vi "Online_Target_2.vi"   [LabVIEW 2021]
uses:
  Model_Updating_Classes/DROPBEAR_Model_Updating/DROPBEAR_Model_Updating.lvclass
types:
  T1 = cluster{"beam_length":dbl, "youngs_modulus":dbl, "torsion_spring":dbl, "beam_height":dbl, "beam_width":dbl, "beam_density":dbl, "number_of_FEA_nodes":i32, "accelerometer_mass":dbl}
  T2 = cluster{"Frequency KF":bool, "Pinned State KF":bool, "FFT Bounding":bool, "Filter Constants Frequency":cluster{"Measurement Variance":dbl, "State Variance":dbl, "Threshold":dbl}, "Filter Constants Position":cluster{"Measurement Variance":dbl, "State Variance":dbl, "Threshold":dbl}, "Moving Window Size":i32, "Time Series buffer":dbl, "Record Time Series Data":bool, "Record Moving Window Data":bool, "Record Online Error Metrics ":bool, "Record Statistics":bool}
  T3 = cluster{"Eigensolver ":enum16{"LabVIEW Cholesky", "LabVIEW General", "LabVIEW Inverse", "LEMP"}, "Models Forcasted":i32, "Max Roller Velocity":dbl, "Max Roller Position Percent":dbl, "Min Roller Position Percent":dbl}
  T4 = cluster{"Dataset":string, "Resample Method":enum16{"Recorded", "Auto Resample", "Custom Resample"}}
  T5 = cluster{"Modeling Parameters input controls":cluster{"beam_length":dbl, "youngs_modulus":dbl, "torsion_spring":dbl, "beam_height":dbl, "beam_width":dbl, "beam_density":dbl, "number_of_FEA_nodes":i32, "accelerometer_mass":dbl}, "Mockbear input controls":cluster{"Dataset":string, "Resample Method":enum16{"Recorded", "Auto Resample", "Custom Resample"}}, "Simulation Parameters input controls":cluster{"Eigensolver ":enum16{"LabVIEW Cholesky", "LabVIEW General", "LabVIEW Inverse", "LEMP"}, "Models Forcasted":i32, "Max Roller Velocity":dbl, "Max Roller Position Percent":dbl, "Min Roller Position Percent":dbl}, "Program Controls":cluster{"Frequency KF":bool, "Pinned State KF":bool, "FFT Bounding":bool, "Filter Constants Frequency":cluster{"Measurement Variance":dbl, "State Variance":dbl, "Threshold":dbl}, "Filter Constants Position":cluster{"Measurement Variance":dbl, "State Variance":dbl, "Threshold":dbl}, "Moving Window Size":i32, "Time Series buffer":dbl, "Record Time Series Data":bool, "Record Moving Window Data":bool, "Record Online Error Metrics ":bool, "Record Statistics":bool}}
  T6 = enum16{"Recorded", "Auto Resample", "Custom Resample"}[]
  T7 = enum16{"LabVIEW Cholesky", "LabVIEW General", "LabVIEW Inverse", "LEMP"}[]
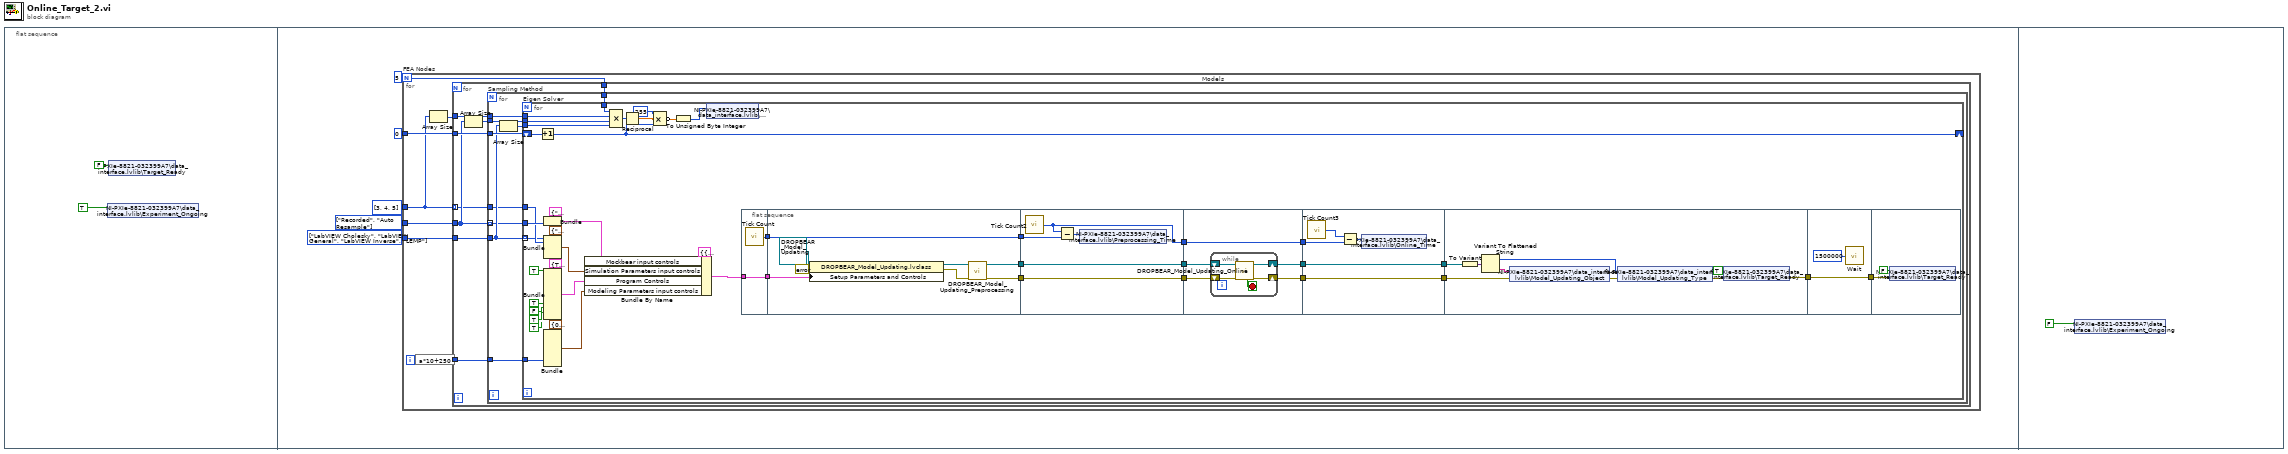
[diagram p0: block diagram]
diagram:
  n1 = flat-sequence {
    frame #0 {
      n2 = shared-variable "NI-PXIe-8821-032399A7\\data_interface.lvlib\\Experiment_Ongoing"(TRUE ("Process_Halt")) -> ()  [unwired: 1 in, 1 out]
      n3 = shared-variable "NI-PXIe-8821-032399A7\\data_interface.lvlib\\Target_Ready"(FALSE ("Target_Ready")) -> ()  [unwired: 1 in, 1 out]
    }
    frame #1 {
      w4 = T6 [enum."Recorded", enum."Auto Resample"] items=["Recorded", "Auto Resample", "Custom Resample"] ("Resample Method")
      w5 = T7 [enum."LabVIEW Cholesky", enum."LabVIEW General", enum."LabVIEW Inverse", enum."LEMP"] items=["LabVIEW Cholesky", "LabVIEW General", "LabVIEW Inverse", "LEMP"] ("Eigensolver")
      n4 = for "FEA Nodes" {
        N: 5 -> [w13]
        tunnel: 0 -> [w12]
        tunnel: w5 -> [w11]
        tunnel: w4 -> [w10]
        tunnel: i32[] [3, 4, 5] -> [w9]
        i -> [w15]
        n5 = expression code="a*10+250"(w15) -> (w14:i32)
        n6 = Array Size(array=w9) -> (size(s)=w8:i32)
        n7 = for "Models" {
          tunnel: w14 -> [w23]
          tunnel: w13 -> [w22]
          tunnel: w12 -> [w21]
          tunnel: w11 -> [w20]
          tunnel: w10 -> [w19]
          tunnel: w9 -> [w17] mode=indexing
          tunnel: w8 -> [w16]
          n8 = Array Size(array=w19) -> (size(s)=w18:i32)
          n9 = for "Sampling Method" {
            tunnel: w23 -> [w32]
            tunnel: w22 -> [w31]
            tunnel: w21 -> [w30]
            tunnel: w20 -> [w28]
            tunnel: w19 -> [w27] mode=indexing
            tunnel: w18 -> [w26]
            tunnel: w17 -> [w25]
            tunnel: w16 -> [w24]
            n10 = Array Size(array=w28) -> (size(s)=w29:i32)
            n11 = for "Eigen Solver" {
              tunnel: w32 -> [w47]
              tunnel: w31 -> [w62]
              shift-right: [w58] -> _
              shift-left: w30 -> [w60]
              tunnel: w28 -> [w33] mode=indexing
              tunnel: w29 -> [w38]
              tunnel: w27 -> [w37]
              tunnel: w26 -> [w36]
              tunnel: w25 -> [w35]
              tunnel: w24 -> [w34]
              n12 = Increment(x=w60) -> (x+1=w58:i32)
              n13 = Bundle(cluster=T4 {"Dataset"="test7", "Resample Method"=enum."Auto Resample"} ("Mockbear input controls"), "Resample Method"=w37) -> (w71:T4)  [unwired: 1 in]
              n14 = Bundle(cluster=T3 {"Eigensolver "=enum."LEMP", "Models Forcasted"=5, "Max Roller Velocity"=3.32, "Max Roller Position Percent"=0.43, "Min Roller Position Percent"=0.155} ("Simulation Parameters input controls"), "Eigensolver"=w33, "Models Forcasted"=w35) -> (w72:T3)  [unwired: 3 in]
              n15 = Bundle(cluster=T2 {"Frequency KF"=TRUE, "Pinned State KF"=FALSE, "FFT Bounding"=FALSE, "Filter Constants Frequency"={"Measurement Variance"=0.4, "State Variance"=0.01, "Threshold"=1000000000.0}, "Filter Constants Position"={"Measurement Variance"=0.4, "State Variance"=0.9, "Threshold"=1000000000.0}, "Moving Window Size"=10, "Time Series buffer"=10000.0, "Record Time Series Data"=FALSE, "Record Moving Window Data"=FALSE, "Record Online Error Metrics "=TRUE, "Record Statistics"=TRUE} ("Program Controls"), "Frequency KF"=TRUE, "Record Time Series Data"=TRUE, "Record Moving Window Data"=FALSE, "Record Online Error Metrics"=TRUE, "Record Statistics"=TRUE) -> (w77:T2)  [unwired: 6 in]
              n16 = Bundle(cluster=T1 {"beam_length"=0.3525, "youngs_modulus"=209500000000.0, "torsion_spring"=0.0, "beam_height"=0.00635, "beam_width"=0.0508, "beam_density"=7900.0, "number_of_FEA_nodes"=40, "accelerometer_mass"=0.055} ("Modeling Parameters input controls"), "number_of_FEA_nodes"=w47) -> (w69:T1)  [unwired: 7 in]
              n17 = Bundle By Name(cluster=T5 {"Modeling Parameters input controls"={"beam_length"=0.3525, "youngs_modulus"=209500000000.0, "torsion_spring"=0.0, "beam_height"=0.00635, "beam_width"=0.0508, "beam_density"=7900.0, "number_of_FEA_nodes"=40, "accelerometer_mass"=0.055}, "Mockbear input controls"={"Dataset"="test7", "Resample Method"=enum."Auto Resample"}, "Simulation Parameters input controls"={"Eigensolver "=enum."LEMP", "Models Forcasted"=5, "Max Roller Velocity"=3.32, "Max Roller Position Percent"=0.43, "Min Roller Position Percent"=0.155}, "Program Controls"={"Frequency KF"=TRUE, "Pinned State KF"=FALSE, "FFT Bounding"=FALSE, "Filter Constants Frequency"={"Measurement Variance"=0.4, "State Variance"=0.01, "Threshold"=1000000000.0}, "Filter Constants Position"={"Measurement Variance"=0.4, "State Variance"=0.9, "Threshold"=1000000000.0}, "Moving Window Size"=10, "Time Series buffer"=10000.0, "Record Time Series Data"=FALSE, "Record Moving Window Data"=FALSE, "Record Online Error Metrics "=TRUE, "Record Statistics"=TRUE}} ("Setup Parameters and Controls"), "Mockbear input controls"=w71, "Simulation Parameters input controls"=w72, "Program Controls"=w77, "Modeling Parameters input controls"=w69) -> (w63:T5)
              n18 = Compound Arithmetic op=MULTIPLY(w62, w34, w36, w38) -> (w61:i32)
              n19 = Reciprocal(x=w61) -> (1/x=w59:dbl)
              n20 = Compound Arithmetic op=MULTIPLY(255, w59, w58) -> (invert w56:dbl)
              n21 = To Unsigned Byte Integer(number=w56) -> (unsigned 8bit integer=w55:u8)
              n22 = shared-variable "NI-PXIe-8821-032399A7\\data_interface.lvlib\\Progress"(w55) -> ()  [unwired: 1 in, 1 out]
              n23 = flat-sequence {
                tunnel: w63 -> [w79]
                tunnel: [w79] -> w50
                tunnel: [w78] -> w48
                tunnel: [w83] -> w54
                tunnel: [w82] -> w52
                tunnel: w50 -> [w81]
                tunnel: [w80] -> w49
                tunnel: w48 -> [w80]
                tunnel: w54 -> [w92]
                tunnel: [w92] -> w53
                tunnel: w52 -> [w91]
                tunnel: [w91] -> w51
                tunnel: w49 -> [w89]
                tunnel: [w88] -> w41
                tunnel: w53 -> [w97]
                tunnel: w51 -> [w96]
                tunnel: [w95] -> w46
                tunnel: [w94] -> w44
                tunnel: [w93] -> w42
                tunnel: w41 -> [w93]
                tunnel: w46 -> [w107]
                tunnel: [w107] -> w45
                tunnel: w44 -> [w106]
                tunnel: [w106] -> w43
                tunnel: w42 -> [w103]
                tunnel: w45 -> [w112]
                tunnel: w43 -> [w111]
                tunnel: [w108] -> w39
                tunnel: [w117] -> w40
                tunnel: w39 -> [w117]
                tunnel: w40 -> [w119]
                frame #0 {
                  n24 = call "Tick Count"() -> ("Tick Count(uSec)"=w78:u32)
                }
                frame #1 {
                  n25 = property class="DROPBEAR_Model_Updating.lvclass"(reference=refnum<class "DROPBEAR_Model_Updating.lvclass"> refnum ("DROPBEAR_Model_Updating.lvclass"), error in=errorcluster {"status"=FALSE, "code"=0, "source"=""} ("error in (no error)"), "Setup Parameters and Controls"=w81) -> (reference out=w87:refnum<class "DROPBEAR_Model_Updating.lvclass">, error out=w84:errorcluster)
                  n26 = call-dynamic "DROPBEAR_Model_Updating_Preprocessing.vi"("error in (no error)"=w84, "DROPBEAR_Model_Updating in"=w87) -> ("error out"=w82:errorcluster, "DROPBEAR_Model_Updating out"=w83:refnum<class "DROPBEAR_Model_Updating.lvclass">)  [unwired: 8 in]
                }
                frame #2 {
                  n27 = call "Tick Count2"() -> ("Tick Count(uSec)"=w88:u32)
                  n28 = Subtract(x=w88, y=w89) -> (x-y=w90:u32)
                  n29 = shared-variable "NI-PXIe-8821-032399A7\\data_interface.lvlib\\Preprocessing_Time"(w90) -> ()  [unwired: 1 in, 1 out]
                }
                frame #3 {
                  n30 = while {
                    shift-right: [w100] -> w95
                    shift-left: w97 -> [w102]
                    shift-right: [w99] -> w94
                    shift-left: w96 -> [w101]
                    stop <- w98 stop-if-true
                    n31 = call-dynamic "DROPBEAR_Model_Updating_Online.vi"("error in (no error)"=w101, "DROPBEAR_Model_Updating in"=w102) -> ("error out"=w99:errorcluster, "DROPBEAR_Model_Updating out"=w100:refnum<class "DROPBEAR_Model_Updating.lvclass">, "looping"=w98:bool)  [unwired: 7 in]
                  }
                }
                frame #4 {
                  n32 = call "Tick Count3"() -> ("Tick Count(uSec)"=w104:u32)
                  n33 = Subtract(x=w104, y=w103) -> (x-y=w105:u32)
                  n34 = shared-variable "NI-PXIe-8821-032399A7\\data_interface.lvlib\\Online_Time"(w105) -> ()  [unwired: 1 in, 1 out]
                }
                frame #5 {
                  n35 = To Variant(anything=w112) -> (Variant=w113:variant)
                  n36 = Variant To Flattened String(Variant=w113) -> (data string=w116:string, 1:w114:i16[])
                  n37 = shared-variable "NI-PXIe-8821-032399A7\\data_interface.lvlib\\Model_Updating_Object"(w116, error in=w111) -> (error out=w115:errorcluster)
                  n38 = shared-variable "NI-PXIe-8821-032399A7\\data_interface.lvlib\\Model_Updating_Type"(w114, error in=w115) -> (error out=w110:errorcluster)
                  n39 = shared-variable "NI-PXIe-8821-032399A7\\data_interface.lvlib\\Target_Ready"(TRUE ("Target_Ready"), error in=w110) -> (error out=w108:errorcluster)
                }
                frame #6 {
                  n40 = call "Wait"("Count(uSec)"=u32 1500000) -> ()  [unwired: 1 out]
                }
                frame #7 {
                  n41 = shared-variable "NI-PXIe-8821-032399A7\\data_interface.lvlib\\Target_Ready"(FALSE ("Target_Ready"), error in=w119) -> ()  [unwired: 1 out]
                }
              }
            }
          }
        }
      }
    }
    frame #2 {
      n42 = shared-variable "NI-PXIe-8821-032399A7\\data_interface.lvlib\\Experiment_Ongoing"(FALSE ("Process_Halt")) -> ()  [unwired: 1 in, 1 out]
    }
  }
